vi "Adjust Application Settings.vi"(8 "error in (no error)":errorcluster, 11 "Application in":refnum<class "Application.lvclass">) -> (0 "error out":errorcluster, 3 "Application out":refnum<class "Application.lvclass">)   [LabVIEW 2017, in "Application.lvlib" / "Application.lvclass"]
doc: "UI used for updating the Settings of an Application. This is a Modal window."
uses:
  Application.lvclass
  <vilib>/TSS/ACRObat Test Framework/Classes/Data/Data Viewer/Settings/Pass Fail Criteria -- Cluster.ctl
  Settings/Class Settings -- Cluster.ctl
  <vilib>/TSS/ACRObat Test Framework/Classes/Data/Data Viewer/Settings/Data Viewer Settings.lvclass
  Settings/App Settings.lvclass
panel:
  in  "Apply":bool
  in  "Cancel":bool
  in  "Close":bool
  in  "Pass Fail Settings":T1
  in  "DataViewer Headers":string[](array[string])
  in  "Meta Values":string[][](array[string])
  in  "Product Name":string
  in  "Test Type":string
  in  "Machine ID":string
  in  "Wait Before Clear":u32 caption="(sec)"
  in  "Cycle Timeout":u32 caption="(sec)"
  in  "AutoClear":bool
  in  "AutoStart":bool
  in  "DataLogging Enabled":bool
  # "DataLogger\nSettings"
  # "Test Application\nSettings"
  # "DataViewer\nSettings"
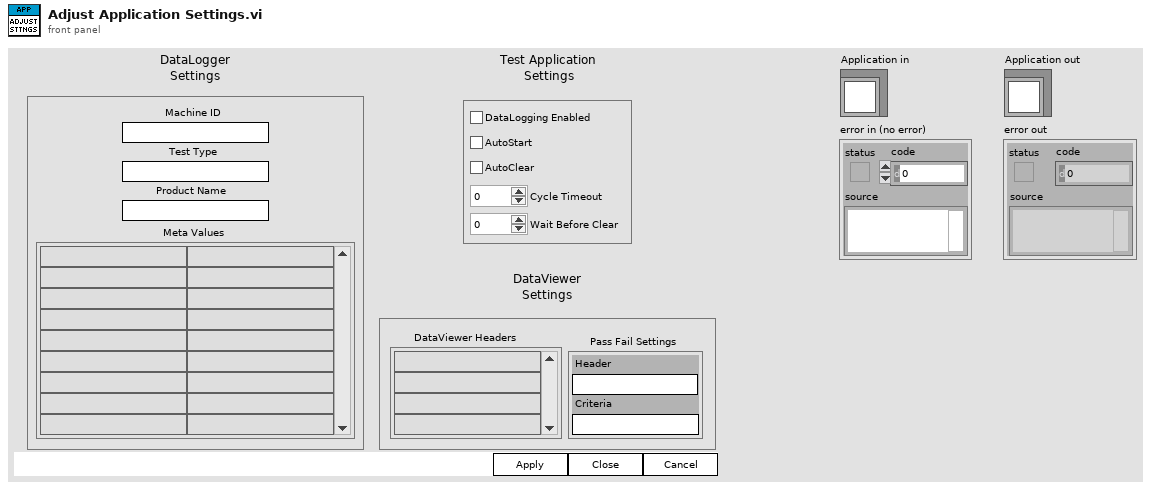
[diagram p1: front panel]
types:
  T1 = typedef "Data Viewer.lvlib/Data Viewer Settings.lvclass/Pass Fail Criteria -- Cluster.ctl" = cluster{"Header":string, "Criteria":string}
  T2 = typedef "Application.lvlib/App Settings.lvclass/Class Settings -- Cluster.ctl" = cluster{"DataLogging Enabled":bool, "AutoStart":bool, "AutoClear":bool, "Cycle Timeout":u32, "Wait Before Clear":u32, "Machine ID":string, "Test Type":string, "Product Name":string, "Meta Tags":string[], "Meta Values":string[], "Viewer Settings":cluster{"DataViewer Headers":string[], "Pass Fail Settings":T1}}
  T3 = cluster{"DataViewer Headers":string[], "Pass Fail Settings":T1}
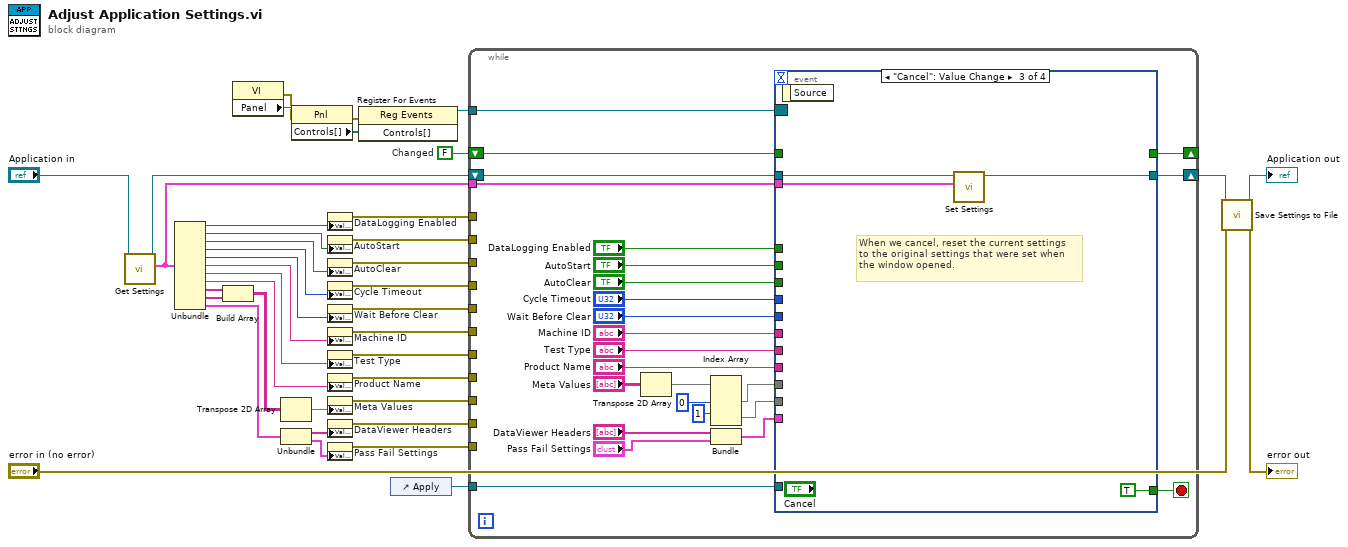
[diagram p0: block diagram]
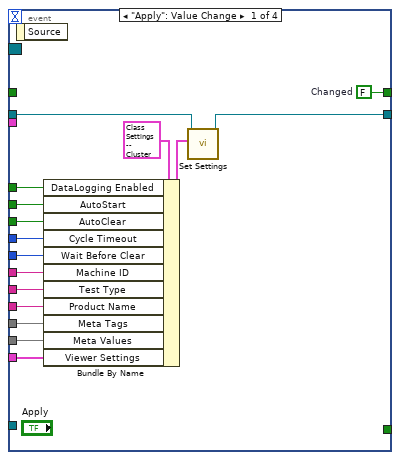
[diagram p2: hidden frame]
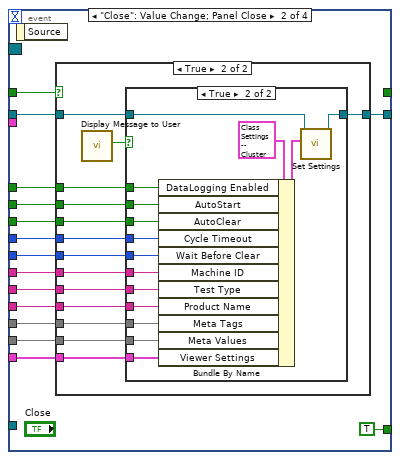
[diagram p3: hidden frame]
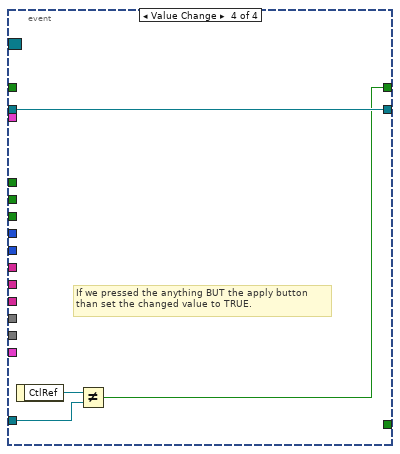
[diagram p6: hidden frame]
diagram:
  w32 = FALSE  # Changed
  n1 = call "Get Settings.vi"("Acrobat Template in"="Application in") -> ("Settings"=w33:T2, "Acrobat Template out"=w34:refnum<class "Application.lvclass">)  [unwired: 8 in, 1 out]
  n2 = Unbundle(w33) -> ("DataLogging Enabled"=w12:bool, "AutoStart"=w11:bool, "AutoClear"=w10:bool, "Cycle Timeout"=w9:u32, "Wait Before Clear"=w8:u32, "Machine ID"=w7:string, "Test Type"=w6:string, "Product Name"=w5:string, "Meta Tags"=w4:string[], "Meta Values"=w3:string[], "Viewer Settings"=w1:T3)
  n3 = Build Array(w4, w3) -> (w2:string[][])
  n4 = property class="VI"() -> (error out=w28:errorcluster, "Panel"=w29:refnum<vi>)  [unwired: 2 in, 1 out]
  n5 = Transpose 2D Array(2D array=w2) -> (transposed array=w13:string[][])
  n6 = Unbundle(w1) -> ("DataViewer Headers"=w36:string[], "Pass Fail Settings"=w35:T1)
  n7 = property class="Pnl"(reference=w29, error in=w28) -> (error out=w31:errorcluster, "Controls[]"=w30:refnum<vi>[])  [unwired: 1 out]
  n8 = property on="DataLogging Enabled" class="Bool (strict)"("Value"=w12) -> (error out=w24:errorcluster)  [unwired: 2 in, 1 out]
  n9 = property on="AutoStart" class="Bool (strict)"("Value"=w11) -> (error out=w23:errorcluster)  [unwired: 2 in, 1 out]
  n10 = property on="AutoClear" class="Bool (strict)"("Value"=w10) -> (error out=w22:errorcluster)  [unwired: 2 in, 1 out]
  n11 = property on="Cycle Timeout" class="DigNum (strict)"("Value"=w9) -> (error out=w21:errorcluster)  [unwired: 2 in, 1 out]
  n12 = property on="Wait Before Clear" class="DigNum (strict)"("Value"=w8) -> (error out=w20:errorcluster)  [unwired: 2 in, 1 out]
  n13 = property on="Machine ID" class="Str"("Value"=w7) -> (error out=w19:errorcluster)  [unwired: 2 in, 1 out]
  n14 = property on="Test Type" class="Str"("Value"=w6) -> (error out=w18:errorcluster)  [unwired: 2 in, 1 out]
  n15 = property on="Product Name" class="Str"("Value"=w5) -> (error out=w17:errorcluster)  [unwired: 2 in, 1 out]
  n16 = property on="Meta Values" class="Arr (strict)"("Value"=w13) -> (error out=w16:errorcluster)  [unwired: 2 in, 1 out]
  n17 = property on="DataViewer Headers" class="Arr (strict)"("Value"=w36) -> (error out=w15:errorcluster)  [unwired: 2 in, 1 out]
  n18 = property on="Pass Fail Settings" class="Clust (strict)"("Value"=w35) -> (error out=w14:errorcluster)  [unwired: 2 in, 1 out]
  n19 = register-events(error in=w31, w30) -> (reference out=w27:refnum<event-registration>)  [unwired: 1 in, 1 out]
  n20 = control-ref of="Apply"() -> (w26:refnum<vi>)
  n21 = while {
    tunnel: w33 -> [w46]
    shift-right: [w47] -> _
    shift-left: w32 -> [w48]
    tunnel: w27 -> [w44]
    shift-right: [w64] -> w38
    shift-left: w34 -> [w65]
    tunnel: w26 -> [w43]
    tunnel: w24 -> [_]
    tunnel: w23 -> [_]
    tunnel: w22 -> [_]
    tunnel: w21 -> [_]
    tunnel: w20 -> [_]
    tunnel: w19 -> [_]
    tunnel: w18 -> [_]
    tunnel: w17 -> [_]
    tunnel: w16 -> [_]
    tunnel: w15 -> [_]
    tunnel: w14 -> [_]
    stop <- w45 stop-if-true
    n22 = Transpose 2D Array(2D array="Meta Values") -> (transposed array=w41:string[][])
    n23 = Index Array(array=w41, index (row) #1=0 ("index (row)"), index (row) #2=1 ("index (row)")) -> (element #1=w51:string[], element #2=w50:string[])  [unwired: 2 in]
    n24 = Bundle("DataViewer Headers"="DataViewer Headers", "Pass Fail Settings"="Pass Fail Settings") -> (w49:T3)  [unwired: 1 in]
    n25 = event shown="[2] \"Cancel\": Value Change" {
      selector: w44 -> [_ _ _ _]
      dyn-events: _ -> [_ _ _ _]
      timeout: _ -> [_ _ _ _]
      tunnel: w65 -> [w81 w96 w131 w135]
      tunnel: [w80 w95 w129 w135] -> w64
      tunnel: "DataLogging Enabled" -> [w74 w91 _ _]
      tunnel: "AutoStart" -> [w73 w90 _ _]
      tunnel: "AutoClear" -> [w72 w89 _ _]
      tunnel: "Cycle Timeout" -> [w71 w88 _ _]
      tunnel: "Wait Before Clear" -> [w70 w87 _ _]
      tunnel: "Machine ID" -> [w69 w86 _ _]
      tunnel: "Test Type" -> [w68 w85 _ _]
      tunnel: "Product Name" -> [w67 w84 _ _]
      tunnel: w51 -> [w77 w94 _ _]
      tunnel: w50 -> [w76 w93 _ _]
      tunnel: w49 -> [w75 w92 _ _]
      tunnel: w48 -> [_ w83 _ _]
      tunnel: [w66 _ _ w132] -> w47
      tunnel: w46 -> [_ _ w130 _]
      tunnel: [_ TRUE TRUE _] -> w45
      tunnel: w43 -> [_ _ _ w134]
      event "Apply": Value Change {
        w66 = FALSE  # Changed
        n26 = event-data() -> ()  [unwired: 1 in, 1 out]
        n27 = Bundle By Name(cluster=T2 {"DataLogging Enabled"=FALSE, "AutoStart"=FALSE, "AutoClear"=FALSE, "Cycle Timeout"=0, "Wait Before Clear"=0, "Machine ID"="", "Test Type"="", "Product Name"="", "Meta Tags"=[], "Meta Values"=[], "Viewer Settings"={"DataViewer Headers"=[], "Pass Fail Settings"={"Header"="", "Criteria"=""}}} ("Settings"), "DataLogging Enabled"=w74, "AutoStart"=w73, "AutoClear"=w72, "Cycle Timeout"=w71, "Wait Before Clear"=w70, "Machine ID"=w69, "Test Type"=w68, "Product Name"=w67, "Meta Tags"=w77, "Meta Values"=w76, "Viewer Settings"=w75) -> (w78:T2)
        n28 = call "Set Settings.vi"("Settings"=w78, "Acrobat Template in"=w81) -> ("Acrobat Template out"=w80:refnum<class "Application.lvclass">)  [unwired: 8 in, 1 out]
      }
      event "Close": Value Change; Panel Close {
        n29 = event-data() -> ()  [unwired: 1 in, 1 out]
        n30 = case shown="True" w83 {
          tunnel: w96 -> [w97 w111]
          tunnel: [w97 w110] -> w95
          tunnel: w94 -> [_ w109]
          tunnel: w93 -> [_ w108]
          tunnel: w92 -> [_ w107]
          tunnel: w91 -> [_ w106]
          tunnel: w90 -> [_ w105]
          tunnel: w89 -> [_ w104]
          tunnel: w88 -> [_ w103]
          tunnel: w87 -> [_ w102]
          tunnel: w86 -> [_ w101]
          tunnel: w85 -> [_ w100]
          tunnel: w84 -> [_ w99]
          frame False {
          }
          frame True {
            n31 = call "Display Message to User"() -> ("OK"=w98:bool)  [unwired: 10 in, 1 out]
            n32 = case shown="True" w98 {
              tunnel: w111 -> [w112 w127]
              tunnel: [w112 w126] -> w110
              tunnel: w109 -> [_ w123]
              tunnel: w108 -> [_ w122]
              tunnel: w107 -> [_ w121]
              tunnel: w106 -> [_ w120]
              tunnel: w105 -> [_ w119]
              tunnel: w104 -> [_ w118]
              tunnel: w103 -> [_ w117]
              tunnel: w102 -> [_ w116]
              tunnel: w101 -> [_ w115]
              tunnel: w100 -> [_ w114]
              tunnel: w99 -> [_ w113]
              frame False {
              }
              frame True {
                n33 = Bundle By Name(cluster=T2 {"DataLogging Enabled"=FALSE, "AutoStart"=FALSE, "AutoClear"=FALSE, "Cycle Timeout"=0, "Wait Before Clear"=0, "Machine ID"="", "Test Type"="", "Product Name"="", "Meta Tags"=[], "Meta Values"=[], "Viewer Settings"={"DataViewer Headers"=[], "Pass Fail Settings"={"Header"="", "Criteria"=""}}} ("Settings"), "DataLogging Enabled"=w120, "AutoStart"=w119, "AutoClear"=w118, "Cycle Timeout"=w117, "Wait Before Clear"=w116, "Machine ID"=w115, "Test Type"=w114, "Product Name"=w113, "Meta Tags"=w123, "Meta Values"=w122, "Viewer Settings"=w121) -> (w124:T2)
                n34 = call "Set Settings.vi"("Settings"=w124, "Acrobat Template in"=w127) -> ("Acrobat Template out"=w126:refnum<class "Application.lvclass">)  [unwired: 8 in, 1 out]
              }
            }
          }
        }
      }
      event "Cancel": Value Change {
        # "When we cancel, reset the current settings\nto the original settings that were set when\nthe window opened."
        n35 = event-data() -> ()  [unwired: 1 in, 1 out]
        n36 = call "Set Settings.vi"("Settings"=w130, "Acrobat Template in"=w131) -> ("Acrobat Template out"=w129:refnum<class "Application.lvclass">)  [unwired: 8 in, 1 out]
      }
      event Value Change {
        # "If we pressed the anything BUT the apply button\nthan set the changed value to TRUE."
        n37 = event-data() -> ("CtlRef"=w133:refnum<vi>)  [unwired: 1 in]
        n38 = Not Equal?(x=w133, y=w134) -> (x != y?=w132:bool)
      }
    }
  }
  n39 = call-dynamic "Save Settings to File.vi"("error in (no error)"="error in (no error)", "Application in"=w38) -> ("error out"=→"error out":errorcluster, "Application out"=→"Application out":refnum<class "Application.lvclass">)  [unwired: 8 in]
